vi "Windowed FFT PtByPt.vi"(0 "x":dbl format="%0.2f", 1 "sample length":i32=100, 2 "window selector":i32(ring) items=["Hanning", "Hamming", "Blackman", "Exact Blackman", "Blackman-Harris"], 4 "initialize":bool) -> (5 "Windowed FFT":cdb[](array[numeric]), 6 "error":i32)   [LabVIEW 2020, in "NI_PtbyPt.lvlib"]
doc: "Computes the windowed fast Fourier transform of the set of input data points specified by <B>sample length</B>."
uses:
  NI_PtbyPt.lvlib
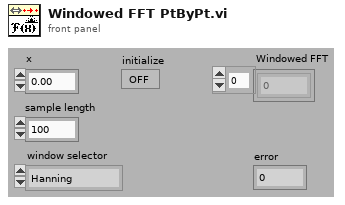
[diagram p1: front panel]
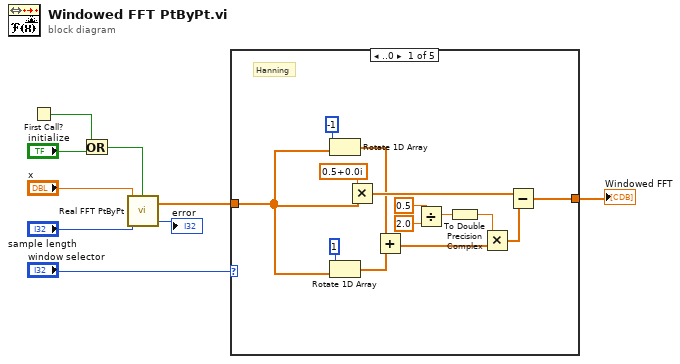
[diagram p0: block diagram]
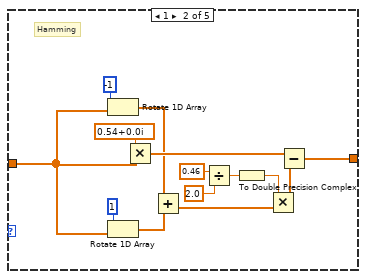
[diagram p2: hidden frame]
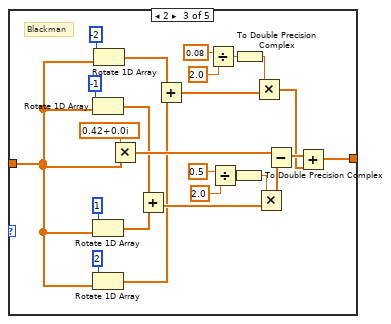
[diagram p3: hidden frame]
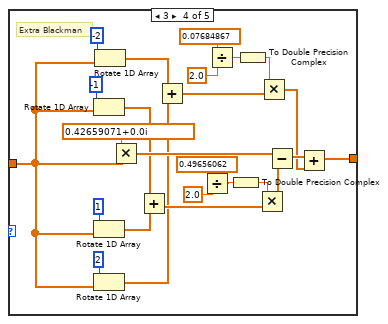
[diagram p4: hidden frame]
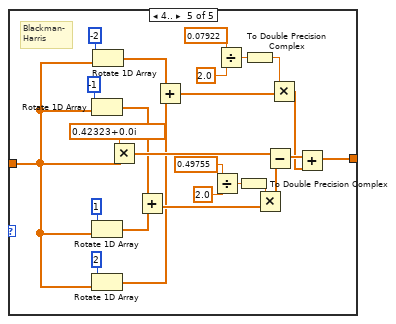
[diagram p5: hidden frame]
diagram:
  n1 = First Call?() -> (First Call?: T/F=w1:bool)
  n2 = Or(x=w1, y="initialize") -> (x .or. y?=w2:bool)
  n3 = call "Real FFT PtByPt.vi"("initialize"=w2, "sample length"="sample length", "x"="x") -> ("error"=→"error":i32, "FFT{X}"=w8:cdb[])  [unwired: 1 in]
  n4 = case shown="..0" "window selector" {
    tunnel: w8 -> [w15 w29 w52 w66 w91]
    tunnel: [w14 w28 w40 w65 w90] -> w7
    frame ..0 {
      # "Hanning"
      n5 = Rotate 1D Array(1:w15, 2:i16 -1 ("n")) -> (0:w19:cdb[])
      n6 = Rotate 1D Array(1:w15, 2:i16 1 ("n")) -> (0:w20:cdb[])
      n7 = Multiply(x=cdb 0.5+0.0i, y=w15) -> (x*y=w22:cdb[])
      n8 = Add(x=w19, y=w20) -> (x+y=w21:cdb[])
      n9 = Divide(x=0.5, y=2.0) -> (x/y=w12:dbl)
      n10 = To Double Precision Complex(1:w12) -> (0:w10:cdb)
      n11 = Multiply(x=w10, y=w21) -> (x*y=w23:cdb[])
      n12 = Subtract(x=w22, y=w23) -> (x-y=w14:cdb[])
    }
    frame 1 {
      # "Hamming"
      n13 = Rotate 1D Array(1:w29, 2:i16 -1 ("n")) -> (0:w33:cdb[])
      n14 = Rotate 1D Array(1:w29, 2:i16 1 ("n")) -> (0:w34:cdb[])
      n15 = Multiply(x=cdb 0.54+0.0i, y=w29) -> (x*y=w36:cdb[])
      n16 = Add(x=w33, y=w34) -> (x+y=w35:cdb[])
      n17 = Divide(x=0.46, y=2.0) -> (x/y=w26:dbl)
      n18 = To Double Precision Complex(1:w26) -> (0:w24:cdb)
      n19 = Multiply(x=w24, y=w35) -> (x*y=w37:cdb[])
      n20 = Subtract(x=w36, y=w37) -> (x-y=w28:cdb[])
    }
    frame 2 {
      # "Blackman"
      n21 = Rotate 1D Array(1:w52, 2:i16 -1 ("n")) -> (0:w58:cdb[])
      n22 = Rotate 1D Array(1:w52, 2:i16 1 ("n")) -> (0:w59:cdb[])
      n23 = Rotate 1D Array(1:w52, 2:i16 2 ("n")) -> (0:w48:cdb[])
      n24 = Rotate 1D Array(1:w52, 2:i16 -2 ("n")) -> (0:w49:cdb[])
      n25 = Multiply(x=cdb 0.42+0.0i, y=w52) -> (x*y=w61:cdb[])
      n26 = Add(x=w58, y=w59) -> (x+y=w60:cdb[])
      n27 = Add(x=w49, y=w48) -> (x+y=w45:cdb[])
      n28 = Divide(x=0.08, y=2.0) -> (x/y=w44:dbl)
      n29 = Divide(x=0.5, y=2.0) -> (x/y=w43:dbl)
      n30 = To Double Precision Complex(1:w43) -> (0:w38:cdb)
      n31 = To Double Precision Complex(1:w44) -> (0:w39:cdb)
      n32 = Multiply(x=w39, y=w45) -> (x*y=w41:cdb[])
      n33 = Multiply(x=w38, y=w60) -> (x*y=w62:cdb[])
      n34 = Subtract(x=w61, y=w62) -> (x-y=w42:cdb[])
      n35 = Add(x=w42, y=w41) -> (x+y=w40:cdb[])
    }
    frame 3 {
      # "Extra Blackman"
      n36 = Rotate 1D Array(1:w66, 2:i16 -1 ("n")) -> (0:w83:cdb[])
      n37 = Rotate 1D Array(1:w66, 2:i16 1 ("n")) -> (0:w84:cdb[])
      n38 = Rotate 1D Array(1:w66, 2:i16 2 ("n")) -> (0:w74:cdb[])
      n39 = Rotate 1D Array(1:w66, 2:i16 -2 ("n")) -> (0:w75:cdb[])
      n40 = Multiply(x=cdb 0.42659071+0.0i, y=w66) -> (x*y=w86:cdb[])
      n41 = Add(x=w83, y=w84) -> (x+y=w85:cdb[])
      n42 = Add(x=w75, y=w74) -> (x+y=w71:cdb[])
      n43 = Divide(x=0.49656062, y=2.0) -> (x/y=w69:dbl)
      n44 = Divide(x=0.07684867, y=2.0) -> (x/y=w70:dbl)
      n45 = To Double Precision Complex(1:w69) -> (0:w63:cdb)
      n46 = To Double Precision Complex(1:w70) -> (0:w64:cdb)
      n47 = Multiply(x=w63, y=w85) -> (x*y=w87:cdb[])
      n48 = Multiply(x=w64, y=w71) -> (x*y=w67:cdb[])
      n49 = Subtract(x=w86, y=w87) -> (x-y=w68:cdb[])
      n50 = Add(x=w68, y=w67) -> (x+y=w65:cdb[])
    }
    frame 4.. {
      # "Blackman-\nHarris"
      n51 = Rotate 1D Array(1:w91, 2:i16 -1 ("n")) -> (0:w108:cdb[])
      n52 = Rotate 1D Array(1:w91, 2:i16 1 ("n")) -> (0:w109:cdb[])
      n53 = Rotate 1D Array(1:w91, 2:i16 2 ("n")) -> (0:w99:cdb[])
      n54 = Rotate 1D Array(1:w91, 2:i16 -2 ("n")) -> (0:w100:cdb[])
      n55 = Multiply(x=cdb 0.42323+0.0i, y=w91) -> (x*y=w111:cdb[])
      n56 = Add(x=w108, y=w109) -> (x+y=w110:cdb[])
      n57 = Add(x=w100, y=w99) -> (x+y=w96:cdb[])
      n58 = Divide(x=0.49755, y=2.0) -> (x/y=w94:dbl)
      n59 = Divide(x=0.07922, y=2.0) -> (x/y=w95:dbl)
      n60 = To Double Precision Complex(1:w94) -> (0:w89:cdb)
      n61 = To Double Precision Complex(1:w95) -> (0:w88:cdb)
      n62 = Multiply(x=w89, y=w110) -> (x*y=w112:cdb[])
      n63 = Subtract(x=w111, y=w112) -> (x-y=w93:cdb[])
      n64 = Multiply(x=w88, y=w96) -> (x*y=w92:cdb[])
      n65 = Add(x=w93, y=w92) -> (x+y=w90:cdb[])
    }
  }
  "Windowed FFT" <- w7
